vi "Config Aout Source.vi"(8 "error in":errorcluster, 9 "Loss (Deviation)":u16(ring) items=["deviation", "bias", "ground"], 10 "Capacitance (Deviation)":u16(ring) items=["deviation", "bias", "ground"], 11 "VISA resource name":refnum<visa-resource-name>) -> (0 "error out":errorcluster, 3 "VISA resource name out":refnum<visa-resource-name>)   [LabVIEW 2019, in "Andeen-Hagerling 2700(400 firmware).lvlib"]
doc: "Selects which analog output voltage source is connected to rear panel analog outputs."
uses:
  Andeen-Hagerling 2700(400 firmware).lvlib
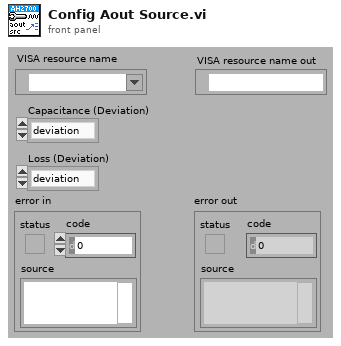
[diagram p1: front panel]
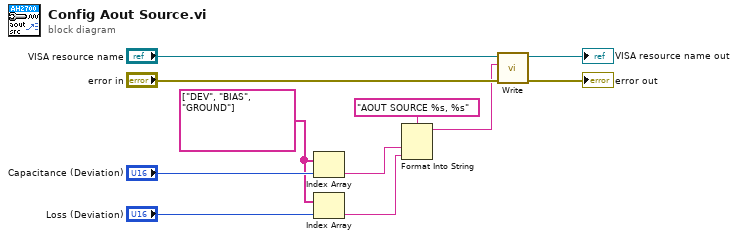
[diagram p0: block diagram]
diagram:
  w4 = string[] ["DEV", "BIAS", "GROUND"]
  n1 = Index Array(array=w4, index="Capacitance (Deviation)") -> (element=w2:string)
  n2 = Index Array(array=w4, index="Loss (Deviation)") -> (element=w1:string)
  n3 = Format Into String(format string="AOUT SOURCE %s, %s", w2, w1) -> (resulting string=w6:string)  [unwired: 2 in, 1 out]
  n4 = call "Write.vi"("error in"="error in", "command"=w6, "VISA resource name"="VISA resource name") -> ("error out"=→"error out":errorcluster, "VISA resource name out"=→"VISA resource name out":refnum<visa-resource-name>)  [unwired: 7 in]
